vi "moving_avg_core.vi"(6 "Array in":dbl[](array[numeric]), 7 "avg":i32, 9 "accumulator in":dbl, 10 "i":i32, 11 "data in":dbl) -> (1 "Array out":dbl[](array[numeric]), 2 "accumulator out":dbl, 3 "rolling avg out":dbl)   [LabVIEW 2011]
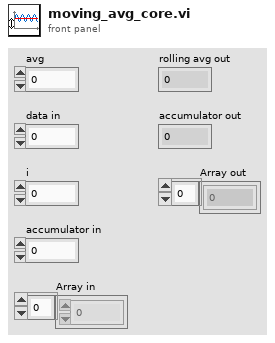
[diagram p1: front panel]
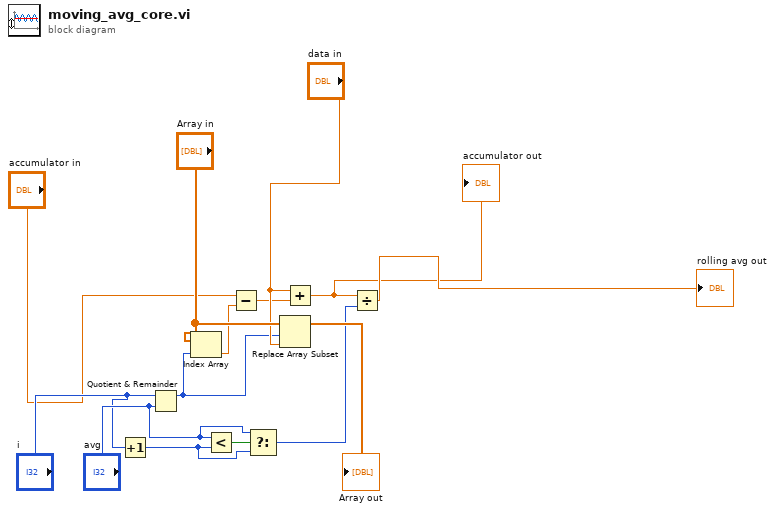
[diagram p0: block diagram]
diagram:
  n1 = Increment(x="i") -> (x+1=w6:i32)
  n2 = Quotient & Remainder(x="i", y="avg") -> (x-y*floor(x/y)=w3:i32)  [unwired: 1 out]
  n3 = Index Array(array="Array in", index=w3) -> (element=w1:dbl)
  n4 = Less?(x="avg", y=w6) -> (x < y?=w4:bool)
  n5 = Subtract(x="accumulator in", y=w1) -> (x-y=w2:dbl)
  n6 = Select(t="avg", s=w4, f=w6) -> (s? t:f=w5:i32)
  n7 = Replace Array Subset(array="Array in", new element="data in", index=w3) -> (→"Array out":dbl[])
  n8 = Add(x="data in", y=w2) -> (x+y=w8:dbl)
  "accumulator out" <- w8
  n9 = Divide(x=w8, y=w5) -> (x/y=→"rolling avg out":dbl)
